vi "LC Global Read VI Controls.vi"(8 "error in (no error)":errorcluster caption="Error In", 9 "Level":i32=1, 10 "vi reference":refnum<vi>, 11 "VI Path":path) -> (0 "error out":errorcluster caption="Error Out")   [LabVIEW 2020]
uses:
  SubVI/LC Mode.ctl
  SubVI/LC Single Control Information.ctl
  SubVI/LC Global Mode.ctl
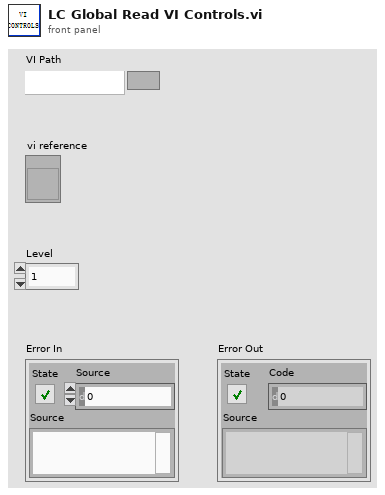
[diagram p1: front panel]
types:
  T1 = typedef "LC Global Mode.ctl" = enum16{"Init", "Read", "Write Language", "Write Version", "Save"}
  T2 = typedef "LC Single Control Information.ctl" = cluster{"VI Path":string, "VI Name":string, "Control Name":string, "Property Type":string, "Language":string, "Content":string}
  T3 = typedef "LC Mode.ctl" = enum16{"Init", "NONE", "Read", "Write", "Delete", "Clear", "Save"}
  T4 = typedef "LC Language Global.ctl" = cluster{"Language":string, "Version":string}
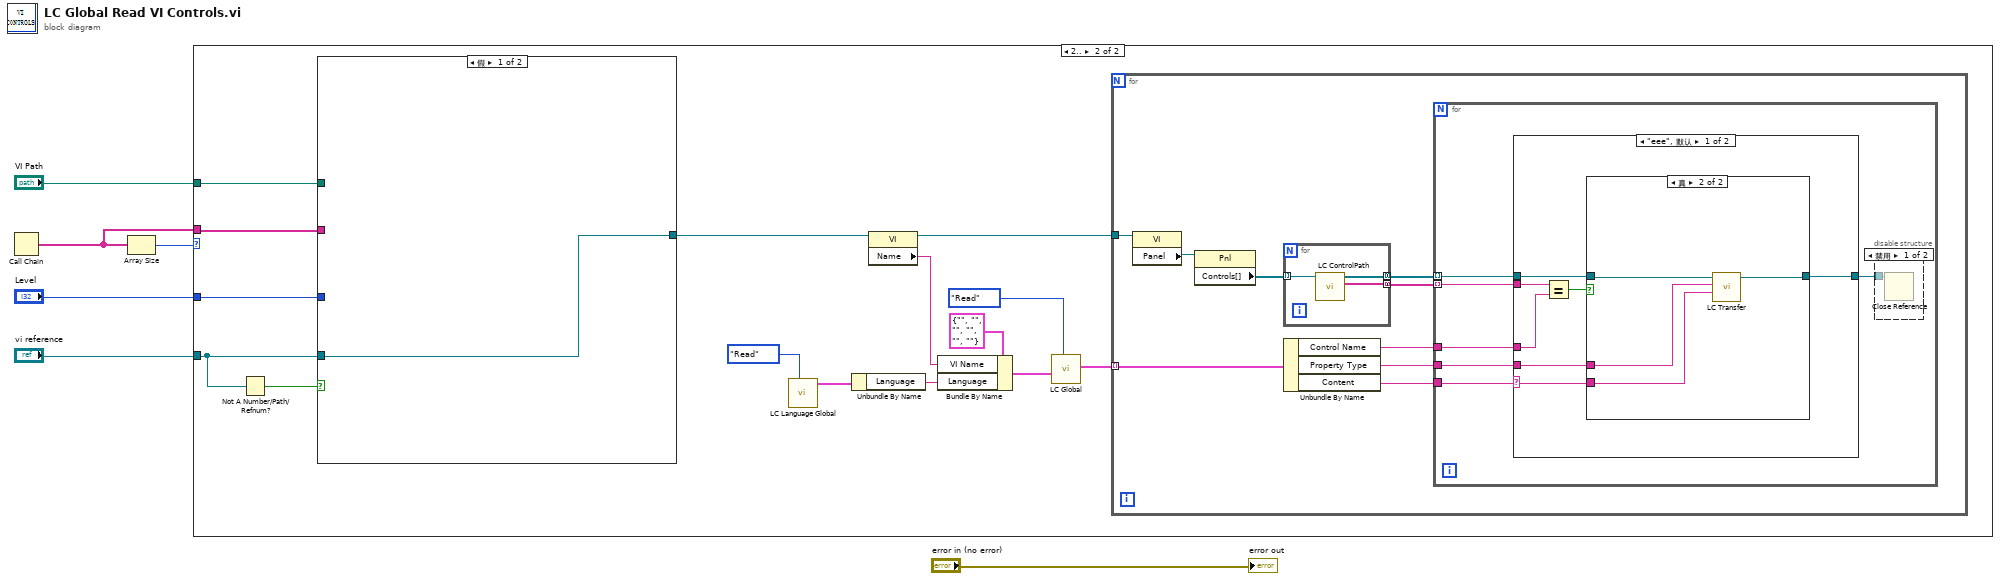
[diagram p0: block diagram]
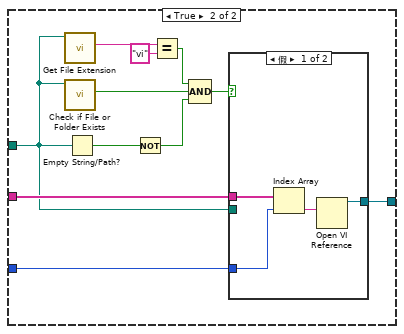
[diagram p3: hidden frame]
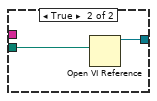
[diagram p4: hidden frame]
diagram:
  n1 = Call Chain() -> (call chain=w5:string[])
  n2 = Array Size(array=w5) -> (size(s)=w6:i32)
  n3 = case shown="2.." w6 {
    tunnel: w5 -> [_ w16]
    tunnel: "VI Path" -> [_ w11]
    tunnel: "Level" -> [_ w9]
    tunnel: "vi reference" -> [_ w7]
    frame 0, Default {
    }
    frame 2.. {
      n4 = Not A Number/Path/Refnum?(number/path/refnum=w7) -> (NaN/Path/Refnum?=w8:bool)
      n5 = case shown="假" w8 {
        tunnel: w16 -> [_ w33]
        tunnel: [w22 w32] -> w15
        tunnel: w11 -> [_ w30]
        tunnel: w9 -> [_ w23]
        tunnel: w7 -> [w22 _]
        frame False {
        }
        frame True {
          n6 = call <vilib>:"Get File Extension.vi"("file"=w30) -> ("lowercase file extension"=w29:string)  [unwired: 6 in, 4 out]
          n7 = call <vilib>:"Check if File or Folder Exists.vi"("path"=w30) -> ("file or folder exists?"=w26:bool)  [unwired: 8 in, 2 out]
          n8 = Empty String/Path?(string/path=w30) -> (empty?=w31:bool)
          n9 = Not(x=w31) -> (.not. x?=w25:bool)
          n10 = Equal?(x=w29, y="vi") -> (x = y?=w27:bool)
          n11 = Compound Arithmetic op=AND ("复合运算")(w27, w26, w25) -> (w24:bool)
          n12 = case shown="假" w24 {
            tunnel: w33 -> [w37 _]
            tunnel: [w35 w38] -> w32
            tunnel: w30 -> [_ w39]
            tunnel: w23 -> [w34 _]
            frame False {
              n13 = Index Array(array=w37, index=w34) -> (element=w36:string)
              n14 = Open VI Reference(vi path=w36) -> (vi reference=w35:refnum<vi>)  [unwired: 5 in, 1 out]
            }
            frame True {
              n15 = Open VI Reference(vi path=w39) -> (vi reference=w38:refnum<vi>)  [unwired: 5 in, 1 out]
            }
          }
        }
      }
      n16 = call "LC Language Global.vi"("Mode"=LC_Global_Mode."Read") -> ("Read"=w18:T4)  [unwired: 9 in, 1 out]
      n17 = Unbundle By Name(w18) -> ("Language"=w17:string)
      n18 = property class="VI"(reference=w15) -> (reference out=w12:refnum<vi>, "Name"=w14:string)  [unwired: 1 in, 1 out]
      n19 = Bundle By Name(cluster=T2 {"VI Path"="", "VI Name"="", "Control Name"="", "Property Type"="", "Language"="", "Content"=""} ("Write"), "VI Name"=w14, "Language"=w17) -> (w19:T2)
      n20 = call "LC Global.vi"("Mode"=LC_Mode."Read", "Write"=w19) -> ("Read"=w13:T2[])  [unwired: 7 in, 2 out]
      n21 = for {
        tunnel: w13 -> [w41] mode=indexing
        tunnel: w12 -> [w48]
        n22 = property class="VI"(reference=w48) -> ("Panel"=w47:refnum<vi>)  [unwired: 1 in, 2 out]
        n23 = property class="Pnl"(reference=w47) -> ("Controls[]"=w46:refnum<vi>[])  [unwired: 1 in, 2 out]
        n24 = for {
          tunnel: w46 -> [w71] mode=indexing
          tunnel: [w70] -> w44 mode=concatenating
          tunnel: [w69] -> w45 mode=concatenating
          n25 = call "LC ControlPath.vi"("Ctl Ref In"=w71) -> ("Control Path Out"=w69:string[], "Ctl Ref Out"=w70:refnum<vi>[])  [unwired: 8 in, 1 out]
        }
        n26 = Unbundle By Name(w41) -> ("Control Name"=w43:string, "Property Type"=w42:string, "Content"=w40:string)
        n27 = for {
          tunnel: w45 -> [w49] mode=indexing
          tunnel: w44 -> [w54] mode=indexing
          tunnel: w43 -> [w50]
          tunnel: w42 -> [w52]
          tunnel: w40 -> [w51]
          n28 = case shown="\"eee\", 默认" w51 {
            selector: w51 -> [w58 _]
            tunnel: w54 -> [w61 w67]
            tunnel: [w60 w67] -> w53
            tunnel: w52 -> [w59 _]
            tunnel: w50 -> [w57 _]
            tunnel: w49 -> [w56 _]
            frame "eee", Default {
              n29 = Equal?(x=w56, y=w57) -> (x = y?=w55:bool)
              n30 = case shown="真" w55 {
                tunnel: w61 -> [w62 w66]
                tunnel: [w62 w65] -> w60
                tunnel: w59 -> [_ w64]
                tunnel: w58 -> [_ w63]
                frame False {
                }
                frame True {
                  n31 = call "LC Transfer.vi"("Value In"=w63, "Property"=w64, "Ctl Ref In"=w66) -> ("Ctl Ref Out"=w65:refnum<vi>)  [unwired: 6 in, 2 out]
                }
              }
            }
            frame "" {
            }
          }
          n32 = disable-structure shown="禁用" {
            disable-tunnel: w53 -> [w68 _]
            frame Disabled {
              n33 = Close Reference(reference=w68) -> ()  [unwired: 1 in, 1 out]
            }
            frame Enabled {
            }
          }
        }
      }
    }
  }
  "error out" <- "error in (no error)"
